vi "0x52_Cmd_read_data_from_a_table_parameter_(SubVI).vi"(10 "Parameters":T1 {"Шаг по данным в словах" min=0 step=4; "Размер поля (слова) в байтах" min=0 step=4; "Размер записываемых данных в байтах" min=0 step=4}, 11 "String in":string) -> (3 "String out":string)   [LabVIEW 2017, in "LV_Unicorn.lvlib"]
uses:
  LV_Unicorn.lvlib
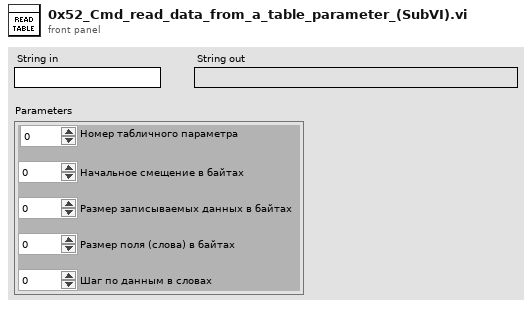
[diagram p1: front panel]
types:
  T1 = cluster{"Начальное смещение в байтах":i32, "Номер табличного параметра":i32, "Размер записываемых данных в байтах":i32, "Размер поля (слова) в байтах":i32, "Шаг по данным в словах":i32}
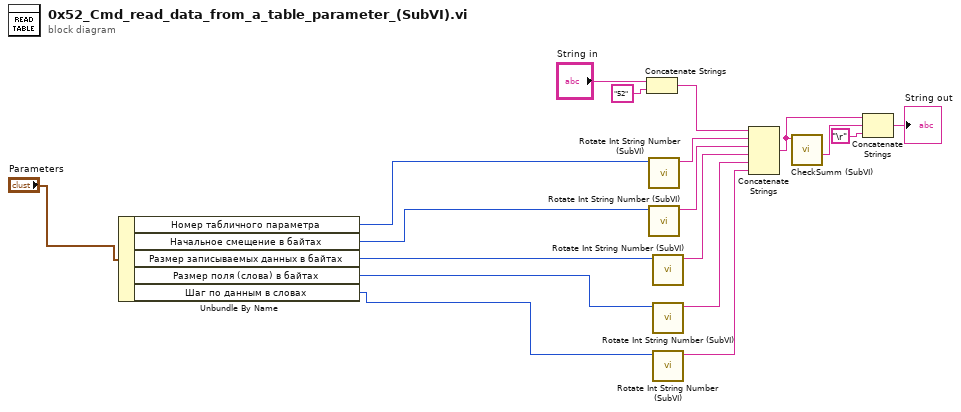
[diagram p0: block diagram]
diagram:
  n1 = Unbundle By Name("Parameters") -> ("Номер табличного параметра"=w8:i32, "Начальное смещение в байтах"=w7:i32, "Размер записываемых данных в байтах"=w5:i32, "Размер поля (слова) в байтах"=w4:i32, "Шаг по данным в словах"=w3:i32)
  n2 = Concatenate Strings("String in", "52" ("string")) -> (w16:string)
  n3 = call "Rotate Int String Number (SubVI).vi"("Int Number In"=w8) -> ("Orig String"=w10:string)  [unwired: 8 in, 2 out]
  n4 = call "Rotate Int String Number (SubVI).vi"("Int Number In"=w7) -> ("Orig String"=w11:string)  [unwired: 8 in, 2 out]
  n5 = call "Rotate Int String Number (SubVI).vi"("Int Number In"=w5) -> ("Orig String"=w9:string)  [unwired: 8 in, 2 out]
  n6 = call "Rotate Int String Number (SubVI).vi"("Int Number In"=w4) -> ("Orig String"=w2:string)  [unwired: 8 in, 2 out]
  n7 = call "Rotate Int String Number (SubVI).vi"("Int Number In"=w3) -> ("Orig String"=w1:string)  [unwired: 8 in, 2 out]
  n8 = Concatenate Strings(w16, w10, w11, w9, w2, w1) -> (w13:string)
  n9 = call "CheckSumm (SubVI).vi"("Input String"=w13) -> ("CheckSumm"=w12:string)  [unwired: 7 in, 3 out]
  n10 = Concatenate Strings(w13, w12, "\r") -> (→"String out":string)
